vi "OFBS_splitTrainingData.vi"(8 "error in (no error)":errorcluster, 9 "Portion of test data":dbl=0.2 format="%#_13g", 10 "Iteration":i32 min=0 max=1 step=1, 11 "OFBS class in":refnum<class "OptFreqBandsSearch.lvclass">) -> (0 "error out":errorcluster, 1 "TestData (cross-check)":cluster{"ClassLabel":string, "Trial":dbl[][]}[](array[cluster]), 2 "TrainData (cross-check)":cluster{"ClassLabel":string, "Trial":dbl[][]}[](array[cluster]), 3 "OFBS class out":refnum<class "OptFreqBandsSearch.lvclass">)   [LabVIEW 2016, in "Optimal Frequency Bands Search.lvlib" / "OptFreqBandsSearch.lvclass"]
doc: "Метод, реализующий чтение обучающих данных (проб) из xml файла"
uses:
  OptFreqBandsSearch.lvclass
  OptFreqBandsSearch.lvclass/OptFreqBandsSearch.ctl
panel:
  # "This VI is a part of BCI Design library, http://www.ru-bci.org \nCopyright © 2020, Sotnikov Peter, All rights reserved. License: CC BY-NC 4.0"
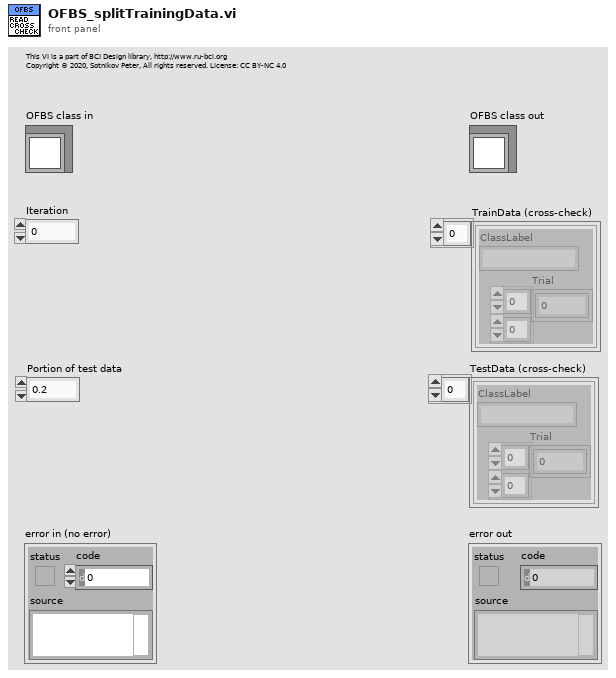
[diagram p1: front panel]
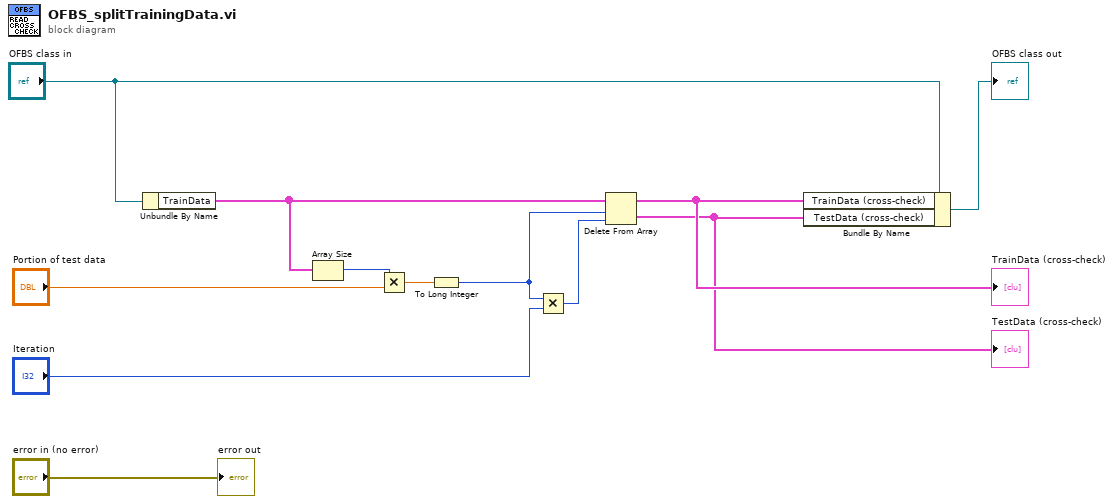
[diagram p0: block diagram]
diagram:
  n1 = Unbundle By Name("OFBS class in") -> ("TrainData"=w3:cluster{"ClassLabel":string, "Trial":dbl[][]}[])
  n2 = Array Size(array=w3) -> (size(s)=w8:i32)
  n3 = Multiply(x=w8, y="Portion of test data") -> (x*y=w9:dbl)
  n4 = To Long Integer(number=w9) -> (32bit integer=w7:i32)
  n5 = Multiply(x=w7, y="Iteration") -> (x*y=w6:i32)
  n6 = Delete From Array(array=w3, length=w7, index=w6) -> (deleted portion=w1:cluster{"ClassLabel":string, "Trial":dbl[][]}[], array with subset deleted=w2:cluster{"ClassLabel":string, "Trial":dbl[][]}[])
  "TrainData (cross-check)" <- w2
  "TestData (cross-check)" <- w1
  n7 = Bundle By Name(cluster="OFBS class in", "TrainData (cross-check)"=w2, "TestData (cross-check)"=w1) -> (→"OFBS class out":refnum<class "OptFreqBandsSearch.lvclass">)
  "error out" <- "error in (no error)"
